vi "Extract Selected Columns.vi"(10 "Visible ML Columns":bool[](array[boolean])=[FALSE, TRUE, TRUE, TRUE, TRUE, TRUE, FALSE, TRUE], 11 "Array in":string[][](array[string])) -> (3 "Selected Columns out":string[][](array[string]))   [LabVIEW 2017, in "Message Log.lvclass"]
uses:
  Message Log.lvclass
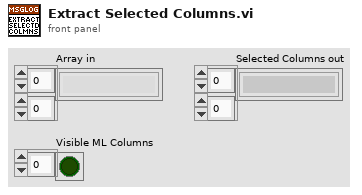
[diagram p1: front panel]
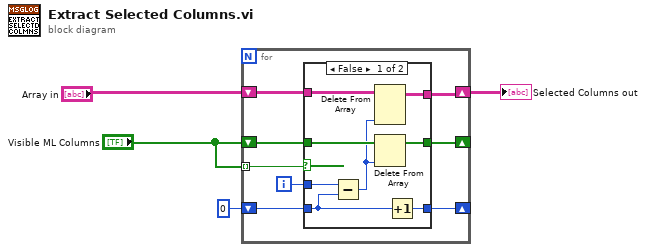
[diagram p0: block diagram]
diagram:
  n1 = for {
    shift-right: [w11] -> w4
    shift-left: "Array in" -> [w12]
    shift-right: [w9] -> _
    shift-left: "Visible ML Columns" -> [w10]
    tunnel: "Visible ML Columns" -> [w8] mode=indexing
    shift-right: [w5] -> _
    shift-left: 0 -> [w6]
    i -> [w7]
    n2 = case shown="False" w8 {
      tunnel: w12 -> [w20 w23]
      tunnel: [w19 w23] -> w11
      tunnel: w10 -> [w18 w22]
      tunnel: [w17 w22] -> w9
      tunnel: w7 -> [w14 _]
      tunnel: w6 -> [w15 w21]
      tunnel: [w16 w21] -> w5
      frame False {
        n3 = Subtract(x=w14, y=w15) -> (x-y=w13:i32)
        n4 = Delete From Array(array=w20, index (col)=w13) -> (array with subset deleted=w19:string[][])  [unwired: 2 in, 1 out]
        n5 = Delete From Array(array=w18, index=w13) -> (array with subset deleted=w17:bool[])  [unwired: 1 in, 1 out]
        n6 = Increment(x=w15) -> (x+1=w16:i32)
      }
      frame True {
      }
    }
  }
  "Selected Columns out" <- w4
